vi "Draw Fill between two plots.vi"(8 "Bottom Line":u32, 9 "Top Line":u32, 10 "Graph Reference":refnum<vi>) -> ()   [LabVIEW 2016, in "Graph Manager.lvclass"]
uses:
  Graph Manager.lvclass
  <vilib>/Analysis/1siggen.llb/Ramp Pattern by Samples.vi
  <vilib>/gmath/NI_Gmath.lvlib
  <vilib>/Analysis/NI_AALBase.lvlib
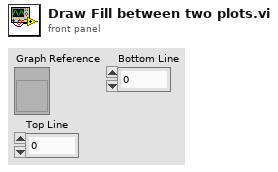
[diagram p1: front panel]
types:
  T1 = typedef "LVBoundsTypeDef.ctl" = cluster{"Width":u32, "Height":u32}
  T2 = typedef "LVRangeTypeDef.ctl" = cluster{"Minimum":dbl, "Maximum":dbl, "Increment":dbl, "Minor Increment":dbl, "Start":dbl}
  T3 = enum32{"Solid", "Dash", "Dot", "DashDot", "DashDotDot"}
  T4 = cluster{i32, "Style":enum32{"Solid", "Dash", "Dot", "DashDot", "DashDotDot"}}
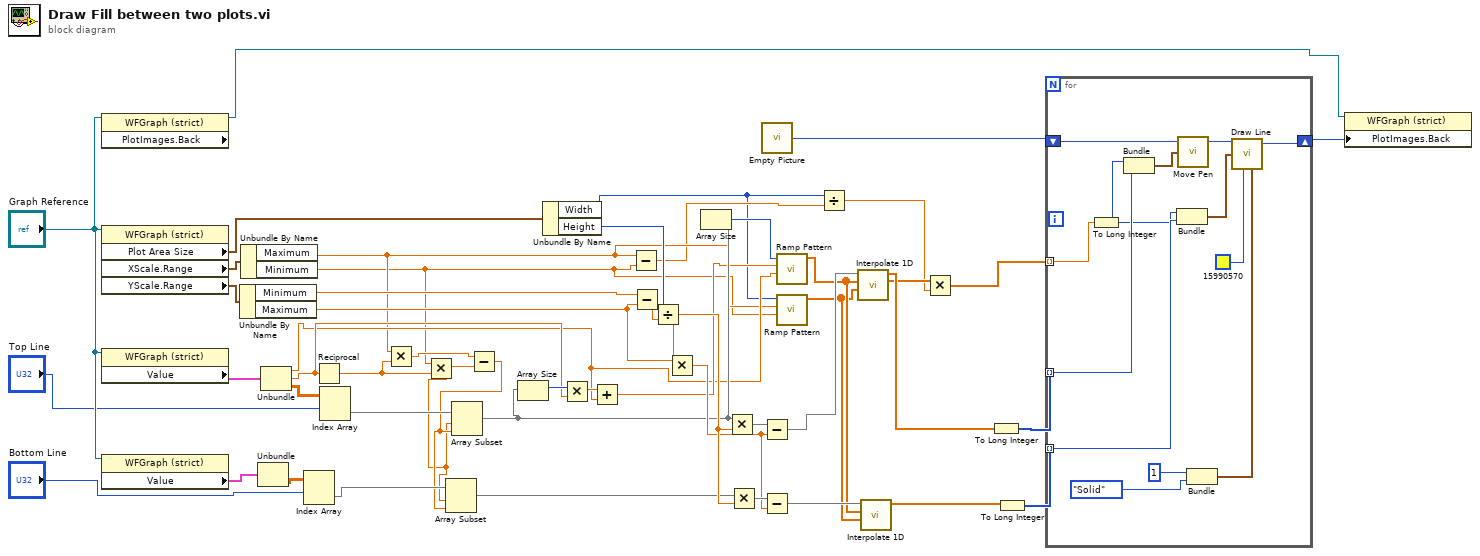
[diagram p0: block diagram]
diagram:
  n1 = property class="WFGraph (strict)" props=["PlotImages.Back"](reference="Graph Reference") -> (reference out=w43:refnum<vi>)  [unwired: 1 in, 2 out]
  n2 = property class="WFGraph (strict)"(reference="Graph Reference") -> ("Plot Area Size"=w47:T1, "XScale.Range"=w32:T2, "YScale.Range"=w33:T2)  [unwired: 1 in, 2 out]
  n3 = property class="WFGraph (strict)"(reference="Graph Reference") -> ("Value"=w25:cluster{dbl, dbl, "Impulses":dbl[][]})  [unwired: 1 in, 2 out]
  n4 = property class="WFGraph (strict)"(reference="Graph Reference") -> ("Value"=w23:cluster{dbl, dbl, "Impulses":dbl[][]})  [unwired: 1 in, 2 out]
  n5 = Unbundle By Name(w33) -> ("Minimum"=w36:dbl, "Maximum"=w35:dbl)
  n6 = Unbundle By Name(w32) -> ("Maximum"=w8:dbl, "Minimum"=w7:dbl)
  n7 = Unbundle(w23) -> ("Impulses"=w22:dbl[][])  [unwired: 2 out]
  n8 = Unbundle(w25) -> (w10:dbl, w13:dbl, "Impulses"=w24:dbl[][])
  n9 = Index Array(array=w22, index (row)="Bottom Line") -> (element=w18:dbl[])  [unwired: 1 in]
  n10 = Reciprocal(x=w13) -> (1/x=w20:dbl)
  n11 = Index Array(array=w24, index (row)="Top Line") -> (element=w21:dbl[])  [unwired: 1 in]
  n12 = Multiply(x=w8, y=w20) -> (x*y=w19:dbl)
  n13 = Multiply(x=w7, y=w20) -> (x*y=w9:dbl)
  n14 = Subtract(x=w19, y=w9) -> (x-y=w16:dbl)
  n15 = Array Subset(array=w18, index=w9, length=w16) -> (w17:dbl[])
  n16 = Array Subset(array=w21, index=w9, length=w16) -> (w14:dbl[])
  n17 = Array Size(array=w14) -> (size(s)=w15:i32)
  n18 = Unbundle By Name(w47) -> ("Width"=w2:u32, "Height"=w38:u32)
  n19 = Multiply(x=w15, y=w13) -> (x*y=w12:dbl)
  n20 = Add(x=w12, y=w10) -> (x+y=w11:dbl)
  n21 = Subtract(x=w8, y=w7) -> (x-y=w3:dbl)
  n22 = Subtract(x=w36, y=w35) -> (x-y=w41:dbl)
  n23 = Divide(x=w38, y=w41) -> (x/y=w40:dbl)
  n24 = Multiply(x=w35, y=w40) -> (x*y=w34:dbl)
  n25 = Array Size(array=w14) -> (size(s)=w4:i32)
  n26 = Multiply(x=w14, y=w40) -> (x*y=w39:dbl[])
  n27 = Multiply(x=w17, y=w40) -> (x*y=w46:dbl[])
  n28 = call "Empty Picture"() -> ("empty picture"=w42:picture)
  n29 = Subtract(x=w39, y=w34) -> (x-y=w31:dbl[])
  n30 = Subtract(x=w46, y=w34) -> (x-y=w29:dbl[])
  n31 = call-poly <vilib>:"Ramp Pattern.vi"("start"=w10, "end"=w11, "samples"=w4) -> ("Ramp Pattern"=w28:dbl[])  [unwired: 7 in, 1 out]
  n32 = call-poly <vilib>:"Ramp Pattern.vi"("start"=w7, "end"=w8, "samples"=w2) -> ("Ramp Pattern"=w27:dbl[])  [unwired: 7 in, 1 out]
  n33 = Divide(x=w2, y=w3) -> (x/y=w5:dbl)
  n34 = call <vilib>:"Interpolate 1D.vi"("xi"=w27, "X"=w28, "Y"=w31) -> ("xi used"=w6:dbl[], "yi"=w30:dbl[])  [unwired: 6 in, 1 out]
  n35 = call <vilib>:"Interpolate 1D.vi"("xi"=w27, "X"=w28, "Y"=w29) -> ("yi"=w26:dbl[])  [unwired: 6 in, 2 out]
  n36 = Multiply(x=w6, y=w5) -> (x*y=w1:dbl[])
  n37 = To Long Integer(number=w30) -> (32bit integer=w37:i32[])
  n38 = To Long Integer(number=w26) -> (32bit integer=w45:i32[])
  n39 = for {
    shift-right: [w60] -> w44
    shift-left: w42 -> [w63]
    tunnel: w37 -> [w62] mode=indexing
    tunnel: w45 -> [w59] mode=indexing
    tunnel: w1 -> [w51] mode=indexing
    n40 = To Long Integer(number=w51) -> (32bit integer=w55:i32)
    n41 = Bundle(w55, "Numeric"=w62) -> (w53:cluster{i32, "Numeric":i32})  [unwired: 1 in]
    n42 = Bundle(w55, "Numeric"=w59) -> (w58:cluster{i32, "Numeric":i32})  [unwired: 1 in]
    n43 = call <vilib>:"Move Pen.vi"("new position"=w53, "picture"=w63) -> ("new picture"=w61:picture)  [unwired: 3 in]
    n44 = Bundle(1, "Style"=T3."Solid") -> (w57:T4)  [unwired: 1 in]
    n45 = call <vilib>:"Draw Line.vi"("picture"=w61, "end point"=w58, "color(black)"=u32 15990570, "pen"=w57) -> ("new picture"=w60:picture)  [unwired: 5 in]
  }
  n46 = property class="WFGraph (strict)"(reference=w43, "PlotImages.Back"=w44) -> ()  [unwired: 1 in, 2 out]
